vi "DailyVideo - ramp up only.vi"() -> ()   [LabVIEW 2020]
panel:
  in  "Current (A) 10":dbl
  in  "Current (A) 9":dbl
  in  "Current (A) 8":dbl
  in  "Current (A) 7":dbl
  in  "Current (A) 6":dbl
  in  "Current (A) 5":dbl
  in  "Current (A) 4":dbl
  in  "Current (A) 3":dbl
  in  "Current (A) 2":dbl
  in  "Time delay between Amp change (s)":dbl
  in  "Channel (1/2)":i32=1
  in  "Current (A)":dbl
  in  "Voltage (V)":dbl
  out "error out":errorcluster
  in  "error in (no error)":errorcluster
  in  "VISA resource name - Instrument Identifier":refnum<visa-resource-name>
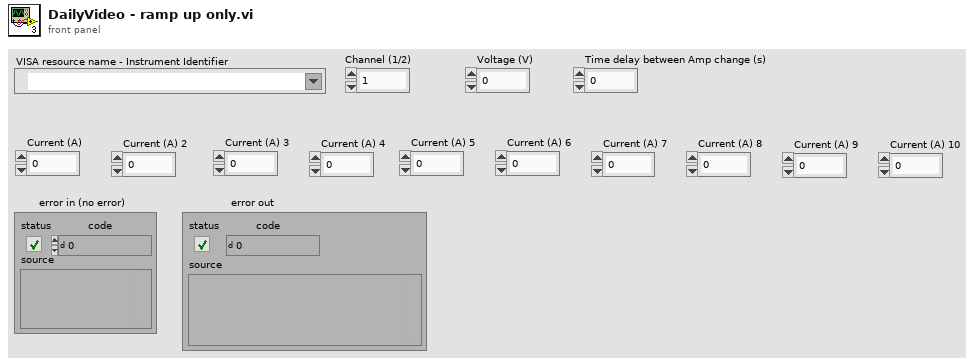
[diagram p1: front panel]
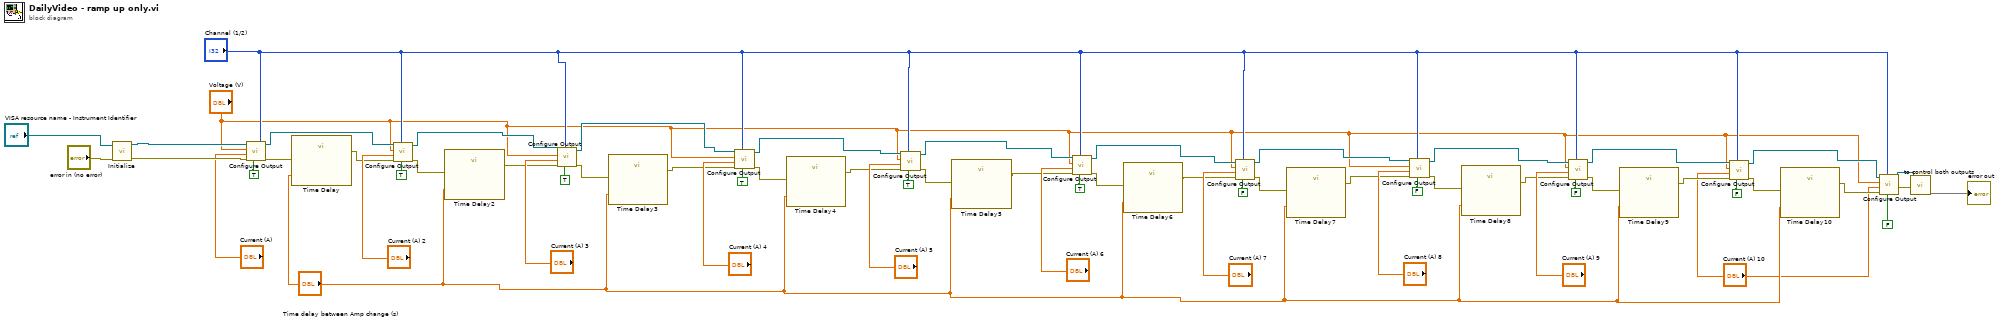
[diagram p0: block diagram]
diagram:
  n1 = call <instrlib>:"Initialize.vi"("error in (no error)"="error in (no error)", "VISA resource name"="VISA resource name - Instrument Identifier") -> ("error out"=w58:errorcluster, "VISA resource name out"=w59:refnum<visa-resource-name>)  [unwired: 8 in]
  n2 = call <instrlib>:"Configure Output.vi"("Enable Output (T: Enable)"=TRUE, "Channel (1:CH1)"="Channel (1/2)", "error in (no error)"=w58, "Current (0 A)"="Current (A)", "Voltage (0 V)"="Voltage (V)", "VISA resource name"=w59) -> ("error out"=w52:errorcluster, "VISA resource name out"=w49:refnum<visa-resource-name>)  [unwired: 4 in]
  n3 = call "Time Delay"("error in (no error)"=w52, "Delay Time (s)"="Time delay between Amp change (s)") -> ("error out"=w48:errorcluster)  [unwired: 9 in]
  n4 = call <instrlib>:"Configure Output.vi"("Enable Output (T: Enable)"=TRUE, "Channel (1:CH1)"="Channel (1/2)", "error in (no error)"=w48, "Current (0 A)"="Current (A) 2", "Voltage (0 V)"="Voltage (V)", "VISA resource name"=w49) -> ("error out"=w47:errorcluster, "VISA resource name out"=w43:refnum<visa-resource-name>)  [unwired: 4 in]
  n5 = call "Time Delay2"("error in (no error)"=w47, "Delay Time (s)"="Time delay between Amp change (s)") -> ("error out"=w42:errorcluster)  [unwired: 9 in]
  n6 = call <instrlib>:"Configure Output.vi"("Enable Output (T: Enable)"=TRUE, "Channel (1:CH1)"="Channel (1/2)", "error in (no error)"=w42, "Current (0 A)"="Current (A) 3", "Voltage (0 V)"="Voltage (V)", "VISA resource name"=w43) -> ("error out"=w44:errorcluster, "VISA resource name out"=w32:refnum<visa-resource-name>)  [unwired: 4 in]
  n7 = call "Time Delay3"("error in (no error)"=w44, "Delay Time (s)"="Time delay between Amp change (s)") -> ("error out"=w31:errorcluster)  [unwired: 9 in]
  n8 = call <instrlib>:"Configure Output.vi"("Enable Output (T: Enable)"=TRUE, "Channel (1:CH1)"="Channel (1/2)", "error in (no error)"=w31, "Current (0 A)"="Current (A) 4", "Voltage (0 V)"="Voltage (V)", "VISA resource name"=w32) -> ("error out"=w39:errorcluster, "VISA resource name out"=w28:refnum<visa-resource-name>)  [unwired: 4 in]
  n9 = call "Time Delay4"("error in (no error)"=w39, "Delay Time (s)"="Time delay between Amp change (s)") -> ("error out"=w27:errorcluster)  [unwired: 9 in]
  n10 = call <instrlib>:"Configure Output.vi"("Enable Output (T: Enable)"=TRUE, "Channel (1:CH1)"="Channel (1/2)", "error in (no error)"=w27, "Current (0 A)"="Current (A) 5", "Voltage (0 V)"="Voltage (V)", "VISA resource name"=w28) -> ("error out"=w36:errorcluster, "VISA resource name out"=w29:refnum<visa-resource-name>)  [unwired: 4 in]
  n11 = call "Time Delay5"("error in (no error)"=w36, "Delay Time (s)"="Time delay between Amp change (s)") -> ("error out"=w30:errorcluster)  [unwired: 9 in]
  n12 = call <instrlib>:"Configure Output.vi"("Enable Output (T: Enable)"=TRUE, "Channel (1:CH1)"="Channel (1/2)", "error in (no error)"=w30, "Current (0 A)"="Current (A) 6", "Voltage (0 V)"="Voltage (V)", "VISA resource name"=w29) -> ("error out"=w33:errorcluster, "VISA resource name out"=w15:refnum<visa-resource-name>)  [unwired: 4 in]
  n13 = call "Time Delay6"("error in (no error)"=w33, "Delay Time (s)"="Time delay between Amp change (s)") -> ("error out"=w14:errorcluster)  [unwired: 9 in]
  n14 = call <instrlib>:"Configure Output.vi"("Enable Output (T: Enable)"=FALSE, "Channel (1:CH1)"="Channel (1/2)", "error in (no error)"=w14, "Current (0 A)"="Current (A) 7", "Voltage (0 V)"="Voltage (V)", "VISA resource name"=w15) -> ("error out"=w24:errorcluster, "VISA resource name out"=w12:refnum<visa-resource-name>)  [unwired: 4 in]
  n15 = call "Time Delay7"("error in (no error)"=w24, "Delay Time (s)"="Time delay between Amp change (s)") -> ("error out"=w8:errorcluster)  [unwired: 9 in]
  n16 = call <instrlib>:"Configure Output.vi"("Enable Output (T: Enable)"=FALSE, "Channel (1:CH1)"="Channel (1/2)", "error in (no error)"=w8, "Current (0 A)"="Current (A) 8", "Voltage (0 V)"="Voltage (V)", "VISA resource name"=w12) -> ("error out"=w21:errorcluster, "VISA resource name out"=w11:refnum<visa-resource-name>)  [unwired: 4 in]
  n17 = call "Time Delay8"("error in (no error)"=w21, "Delay Time (s)"="Time delay between Amp change (s)") -> ("error out"=w7:errorcluster)  [unwired: 9 in]
  n18 = call <instrlib>:"Configure Output.vi"("Enable Output (T: Enable)"=FALSE, "Channel (1:CH1)"="Channel (1/2)", "error in (no error)"=w7, "Current (0 A)"="Current (A) 9", "Voltage (0 V)"="Voltage (V)", "VISA resource name"=w11) -> ("error out"=w18:errorcluster, "VISA resource name out"=w10:refnum<visa-resource-name>)  [unwired: 4 in]
  n19 = call "Time Delay9"("error in (no error)"=w18, "Delay Time (s)"="Time delay between Amp change (s)") -> ("error out"=w6:errorcluster)  [unwired: 9 in]
  n20 = call <instrlib>:"Configure Output.vi"("Enable Output (T: Enable)"=FALSE, "Channel (1:CH1)"="Channel (1/2)", "error in (no error)"=w6, "Current (0 A)"="Current (A) 10", "Voltage (0 V)"="Voltage (V)", "VISA resource name"=w10) -> ("error out"=w16:errorcluster, "VISA resource name out"=w9:refnum<visa-resource-name>)  [unwired: 4 in]
  n21 = call "Time Delay10"("error in (no error)"=w16, "Delay Time (s)"="Time delay between Amp change (s)") -> ("error out"=w5:errorcluster)  [unwired: 9 in]
  n22 = call <instrlib>:"Configure Output.vi"("Enable Output (T: Enable)"=FALSE, "Channel (1:CH1)"="Channel (1/2)", "error in (no error)"=w5, "Current (0 A)"="Current (A) 10", "Voltage (0 V)"="Voltage (V)", "VISA resource name"=w9) -> ("error out"=w4:errorcluster, "VISA resource name out"=w57:refnum<visa-resource-name>)  [unwired: 4 in]
  n23 = call "to control both outputs.vi"(8:w4, 11:w57) -> (0:→"error out")  [unwired: 9 in]
